vi "GetRingReference.vi"(8 "error in":errorcluster, 11 "Ring in":refnum<class "Ring.lvclass">) -> (0 "error out":errorcluster, 1 "Ring reference":refnum<vi>, 3 "Ring out":refnum<class "Ring.lvclass">)   [LabVIEW 2014, in "Raspberry Pi Compatible Compiler for LabVIEW.lvlib" / "Ring.lvclass"]
uses:
  Ring.lvclass
  Generic/Generic.lvclass
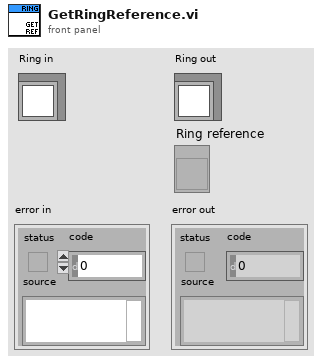
[diagram p1: front panel]
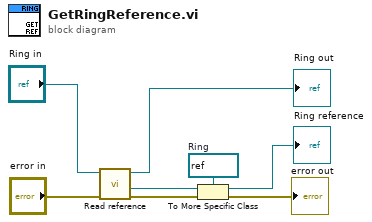
[diagram p0: block diagram]
diagram:
  w6 = refnum<vi> refnum  # Ring
  n1 = call "Read reference.vi"("error in"="error in", "GObject in"="Ring in") -> ("error out"=w7:errorcluster, "reference"=w8:refnum<vi>, "GObject out"=→"Ring out":refnum<class "Ring.lvclass">)  [unwired: 5 in]
  n2 = To More Specific Class(target class=w6, reference=w8, error in=w7) -> (specific class reference=→"Ring reference":refnum<vi>, error out=→"error out":errorcluster)
